vi "Initialize.vi"(8 "error in (no error)":errorcluster, 9 "Reset (T: Reset)":bool=TRUE, 10 "ID Query (T: Check)":bool=TRUE, 11 "VISA Resource Name":refnum<visa-resource-name>) -> (0 "error out":errorcluster, 3 "VISA Resource Name Out":refnum<visa-resource-name> caption="VISA session")   [LabVIEW 2010, in "Stanford Research 844.lvlib"]
doc: "This VI passes the addressing information in the instrument descriptor to the Instr Open VI and returns the instrument ID. You can optionally reset the instrument by setting the front panel reset control. You must run this VI before using any of the instrument driver VIs for this instrument.\n\nNote:\nIf you are using serial interface to communicate with your instrument, make sure the VISA COM port settings on your PC match the COM port settings on the instrument.\n\nTo check the VISA COM port settings launch Measurement&Automation Explorer and go to Devices and Interfaces > Ports, right-click on the COM port you want to use and select Properties. Here go to tab Port Settings.\n\nTo check the COM port settings on the instrument, refer to the operating manual."
uses:
  <instrlib>/Stanford Research 844/Stanford Research 844.lvlib
panel:
  # "© 2005 National Instruments.  ALL RIGHTS RESERVED."
  # "If you are using serial interface to communicate\nwith your instrument, read note in the \nVI Properties > Documentation."
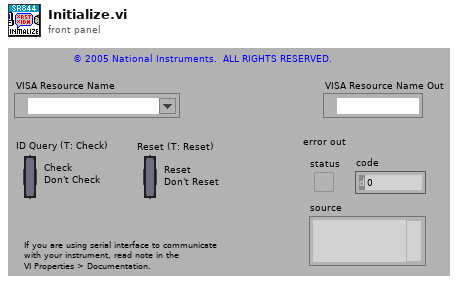
[diagram p1: front panel]
types:
  T1 = cluster{"status":bool, "code":i32, "regular expression":string}
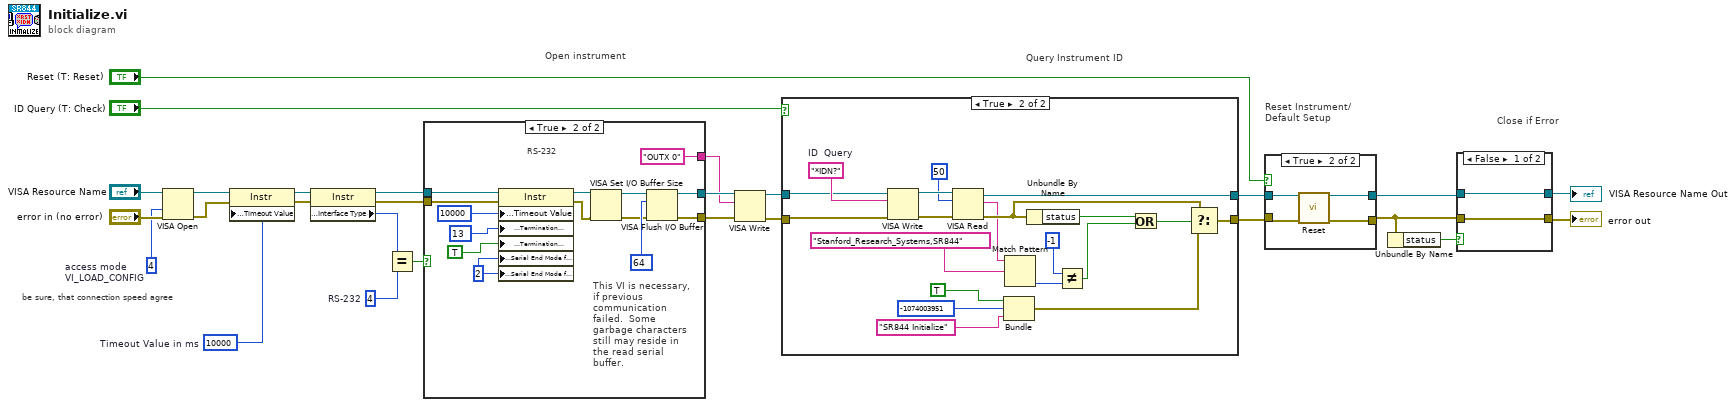
[diagram p0: block diagram]
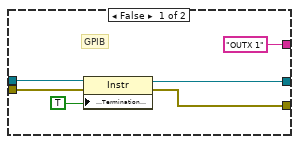
[diagram p2: hidden frame]
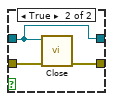
[diagram p3: hidden frame]
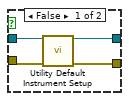
[diagram p4: hidden frame]
diagram:
  w21 = u16 4  # RS-232
  w10 = u32 4  # access mode VI_LOAD_CONFIG
  w8 = u32 10000  # Timeout Value in ms
  # "be sure, that connection speed agree"
  # "Close if Error"
  # "Query Instrument ID"
  # "Reset Instrument/\nDefault Setup"
  # "Open instrument"
  n1 = VISA Open(access mode=w10, error in (no error)="error in (no error)", VISA resource name="VISA Resource Name") -> (VISA resource name=w7:refnum<visa-resource-name>, error out=w6:errorcluster)  [unwired: 2 in]
  n2 = property class="Instr"(reference=w7, error in=w6, "General Settings:Timeout Value"=w8) -> (reference out=w24:refnum<visa-resource-name>, error out=w23:errorcluster)
  n3 = property class="Instr"(reference=w24, error in=w23) -> (reference out=w13:refnum<visa-resource-name>, error out=w12:errorcluster, "Interface Information:Interface Type"=w22:u16)
  n4 = Equal?(x=w22, y=w21) -> (x = y?=w20:bool)
  n5 = case shown="True" w20 {
    tunnel: w13 -> [w33 w38]
    tunnel: w12 -> [w32 w37]
    tunnel: [w31 w44] -> w4
    tunnel: [w30 w43] -> w3
    tunnel: ["OUTX 1" "OUTX 0"] -> w1
    frame False {
      # "GPIB"
      n6 = property class="Instr"(reference=w33, error in=w32, "Message Based Settings:Termination Character Enable"=TRUE) -> (reference out=w31:refnum<visa-resource-name>, error out=w30:errorcluster)
    }
    frame True {
      w39 = u16 2 ("ASRL End In")
      # "RS-232"
      # "This VI is necessary, if previous communication failed.  Some garbage characters still may reside in the read serial buffer."
      n7 = property class="Instr"(reference=w38, error in=w37, "General Settings:Timeout Value"=u32 10000, "Message Based Settings:Termination Character"=u8 13 ("TermChar"), "Message Based Settings:Termination Character Enable"=TRUE ("TermChar En"), "Serial Settings:Serial End Mode for Reads"=w39, "Serial Settings:Serial End Mode for Writes"=w39) -> (reference out=w36:refnum<visa-resource-name>, error out=w35:errorcluster)
      n8 = VISA Set I/O Buffer Size(VISA resource name=w36, error in (no error)=w35) -> (VISA resource name out=w46:refnum<visa-resource-name>, error out=w45:errorcluster)  [unwired: 2 in]
      n9 = VISA Flush I/O Buffer(VISA resource name=w46, mask (16)=u16 64 ("Serial Settings:Serial End Mode for Writes"), error in (no error)=w45) -> (VISA resource name out=w44:refnum<visa-resource-name>, error out=w43:errorcluster)
    }
  }
  n10 = VISA Write(VISA resource name=w4, write buffer=w1, error in (no error)=w3) -> (VISA resource name out=w5:refnum<visa-resource-name>, error out=w2:errorcluster)  [unwired: 1 out]
  n11 = case shown="True" "ID Query (T: Check)" {
    tunnel: [w48 w50] -> w17
    tunnel: [w49 w51] -> w16
    tunnel: w5 -> [w49 w53]
    tunnel: w2 -> [w48 w52]
    frame False {
    }
    frame True {
      w67 = "*IDN?"  # ID  Query
      n12 = VISA Write(VISA resource name=w53, write buffer=w67, error in (no error)=w52) -> (VISA resource name out=w69:refnum<visa-resource-name>, error out=w68:errorcluster)  [unwired: 1 out]
      n13 = VISA Read(VISA resource name=w69, byte count=u32 50 ("byte count (0)"), error in (no error)=w68) -> (VISA resource name out=w51:refnum<visa-resource-name>, read buffer=w62:string, error out=w65:errorcluster)  [unwired: 1 out]
      n14 = Bundle(TRUE, -1074003951, "regular expression"="SR844 Initialize") -> (w57:cluster{bool, i32, "regular expression":string})  [unwired: 1 in]
      n15 = Match Pattern(string=w62, regular expression="Stanford_Research_Systems,SR844") -> (offset past match=w60:i32)  [unwired: 1 in, 3 out]
      n16 = Unbundle By Name(w65) -> ("status"=w64:bool)
      n17 = Not Equal?(x=-1, y=w60) -> (x != y?=w58:bool)
      n18 = Or(x=w64, y=w58) -> (x .or. y?=w63:bool)
      n19 = Select(t=w65, s=w63, f=w57) -> (s? t:f=w50:T1)
    }
  }
  n20 = case shown="True" "Reset (T: Reset)" {
    tunnel: w17 -> [w72 w75]
    tunnel: [w70 w77] -> w18
    tunnel: w16 -> [w73 w76]
    tunnel: [w71 w74] -> w19
    frame False {
      n21 = call <instrlib>:"Utility Default Instrument Setup.vi"("VISA Resource Name"=w73, "error in (no error)"=w72) -> ("VISA Resource Name Out"=w71:refnum<visa-resource-name>, "error out"=w70:errorcluster)  [unwired: 12 in]
    }
    frame True {
      n22 = call <instrlib>:"Reset.vi"("VISA Resource Name"=w76, "error in (no error)"=w75) -> ("VISA Resource Name Out"=w74:refnum<visa-resource-name>, "error out"=w77:errorcluster)  [unwired: 12 in]
    }
  }
  n23 = Unbundle By Name(w18) -> ("status"=w25:bool)
  n24 = case shown="False" w25 {
    tunnel: w19 -> [w79 w80]
    tunnel: w18 -> [w78 w81]
    tunnel: [w79 w80] -> w15
    tunnel: [w78 w82] -> w14
    frame False {
    }
    frame True {
      n25 = call <instrlib>:"Close.vi"("error in (no error)"=w81, "VISA Resource Name"=w80) -> ("error out"=w82:errorcluster)  [unwired: 9 in]
    }
  }
  "error out" <- w14
  "VISA Resource Name Out" <- w15
